vi "Send VHM-setSettings.vi"(7 "Message Priority (Normal)":T3=enum."Normal", 8 "error in (no error)":errorcluster, 10 "settings":T1={"Start [hz]"=0, "Stop [hz]"=0, "sampleSize"=101} {"sampleSize" items=["101"=101, "201"=201, "401"=401, "601"=601, "801"=801, "1001"=1001]; "Stop [hz]" format="%.0p"; "Start [hz]" format="%.0p"}, 11 "Message Enqueuer":refnum<class "Message Enqueuer.lvclass">) -> (0 "error out":errorcluster, 3 "Message Enqueuer out":refnum<class "Message Enqueuer.lvclass">)   [LabVIEW 2020, in "VHM-VNA_Hardware_Manager.lvlib" / "VHM-setSettings Msg.lvclass"]
doc: "This VI sends the message to an actor."
uses:
  VHM-setSettings Msg.lvclass
  <vilib>/ActorFramework/Message Enqueuer/Message Enqueuer.lvclass
  <vilib>/ActorFramework/Message Enqueuer/Message Priority.ctl
  classes/vna-drivers/liteVNA/VD-settingsEasy.ctl
  classes/vna-drivers/liteVNA/VD-sampleSize.ctl
  C:/Program Files (x86)/National Instruments/LabVIEW 2020/vi.lib/ActorFramework/Message/Message.lvclass
  VHM-setSettings Msg.lvclass/VHM-setSettings Msg.ctl
  <vilib>/ActorFramework/Message Enqueuer/Message Enqueuer.lvclass/Message Enqueuer.ctl
  <vilib>/ActorFramework/Message Priority Queue/Priority Enqueue.vi
  classes/vna-drivers/liteVNA/VD-LV-LiteVNA.lvclass
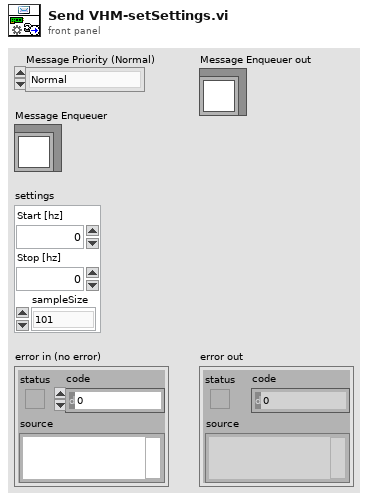
[diagram p1: front panel]
types:
  T1 = typedef "VD-LV-LiteVNA.lvclass/VD-settingsEasy.ctl" = cluster{"Start [hz]":u64, "Stop [hz]":u64, "sampleSize":T2}
  T2 = typedef "VD-LV-LiteVNA.lvclass/VD-sampleSize.ctl" = u16
  T3 = typedef "Actor Framework.lvlib/Message Enqueuer.lvclass/Message Priority.ctl" = enum16{"Low", "Normal", "High"}
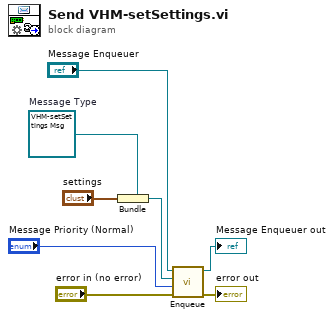
[diagram p0: block diagram]
diagram:
  w5 = refnum<class "VHM-setSettings Msg.lvclass"> refnum  # Message Type
  n1 = Bundle(cluster=w5, "settings") -> (w4:refnum<class "VHM-setSettings Msg.lvclass">)
  n2 = call <vilib>:"Enqueue.vi"("error in (no error)"="error in (no error)", "Message Priority (Normal)"="Message Priority (Normal)", "Message"=w4, "Message Enqueuer in"="Message Enqueuer") -> ("error out"=→"error out":errorcluster, "Message Enqueuer out"=→"Message Enqueuer out":refnum<class "Message Enqueuer.lvclass">)  [unwired: 6 in]
